vi "全局 1.vi"() -> ()   [LabVIEW 2015]
panel:
  in  "停止":bool
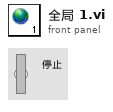
[diagram p1: front panel]
diagram:
